vi "Solenoids_and_Deflection.vi"() -> ()   [LabVIEW 2018]
panel:
  out "?":string
  out "?":string
  out "?":string
  out "?":string
  in  "Set Agilent 2":bool
  out "?":bool
  out "?":bool
  out "?":string
  in  "Set Agilent":bool
  out "?":bool
  out "?":bool
  out "?":string
  out "Sensors":string
  # "Waveform:\nTriangle"
  # "Peak B-Field:\n90 G"
  # "Solenoid (M1)"
  # "Freq | Amp:\n20 Hz | 10 V"
  # "Peak Current:\n1.7 A"
  # "Solenoid (M2)"
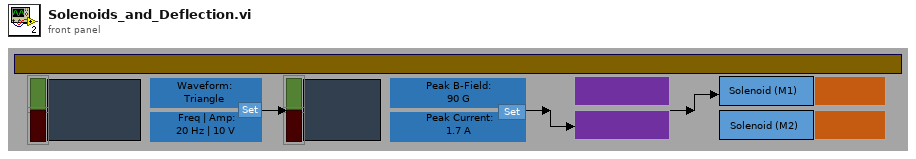
[diagram p1: front panel]
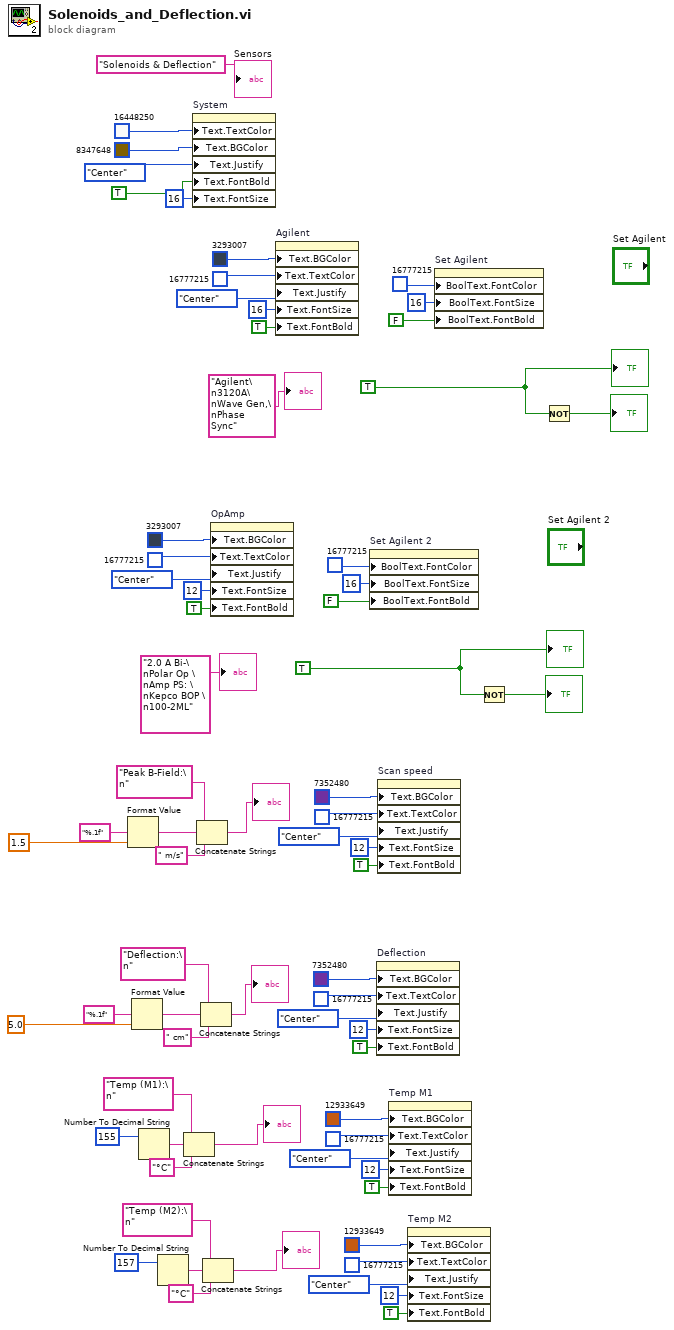
[diagram p0: block diagram]
diagram:
  w44 = TRUE
  w55 = TRUE
  n1 = Format Value(format string="%.1f", value (0)=1.5) -> (output string=w29:string)  [unwired: 1 in]
  n2 = Format Value(format string="%.1f", value (0)=5.0) -> (output string=w23:string)  [unwired: 1 in]
  n3 = Number To Decimal String(number=155) -> (decimal integer string=w14:string)  [unwired: 1 in]
  n4 = Number To Decimal String(number=157) -> (decimal integer string=w4:string)  [unwired: 1 in]
  n5 = Concatenate Strings("Temp (M1):\n", w14, "°C" ("string")) -> (→"?":string)
  n6 = property on="System" class="Str"("Text.TextColor"=u32 16448250, "Text.BGColor"=u32 8347648, "Text.Justify"=enum16{"Left", "Center", "Right"}."Center" ("Text.Justification"), "Text.FontBold"=TRUE ("Text.Font:Bold"), "Text.FontSize"=u32 16 ("Text.Font:Size")) -> ()  [unwired: 2 in, 2 out]
  n7 = Concatenate Strings("Peak B-Field:\n", w29, " m/s" ("string")) -> (→"?":string)
  n8 = Concatenate Strings("Deflection:\n", w23, " cm" ("string")) -> (→"?":string)
  n9 = Concatenate Strings("Temp (M2):\n", w4, "°C" ("string")) -> (→"?":string)
  n10 = property on="OpAmp" class="Str"("Text.BGColor"=u32 3293007, "Text.TextColor"=u32 16777215, "Text.Justify"=enum16{"Left", "Center", "Right"}."Center" ("Text.Justification"), "Text.FontSize"=u32 12 ("Text.Font:Size"), "Text.FontBold"=TRUE ("Text.Font:Bold")) -> ()  [unwired: 2 in, 2 out]
  n11 = property on="Agilent" class="Str"("Text.BGColor"=u32 3293007, "Text.TextColor"=u32 16777215, "Text.Justify"=enum16{"Left", "Center", "Right"}."Center" ("Text.Justification"), "Text.FontSize"=u32 16 ("Text.Font:Size"), "Text.FontBold"=TRUE ("Text.Font:Bold")) -> ()  [unwired: 2 in, 2 out]
  n12 = property on="Set Agilent 2" class="Bool (strict)"("BoolText.FontColor"=u32 16777215, "BoolText.FontSize"=u32 16 ("Boolean Text.Font:Size"), "BoolText.FontBold"=FALSE ("Boolean Text.Font:Bold")) -> ()  [unwired: 2 in, 2 out]
  n13 = property on="Deflection" class="Str"("Text.BGColor"=u32 7352480, "Text.TextColor"=u32 16777215, "Text.Justify"=enum16{"Left", "Center", "Right"}."Center" ("Text.Justification"), "Text.FontSize"=u32 12 ("Text.Font:Size"), "Text.FontBold"=TRUE ("Text.Font:Bold")) -> ()  [unwired: 2 in, 2 out]
  n14 = property on="Scan speed" class="Str"("Text.BGColor"=u32 7352480, "Text.TextColor"=u32 16777215, "Text.Justify"=enum16{"Left", "Center", "Right"}."Center" ("Text.Justification"), "Text.FontSize"=u32 12 ("Text.Font:Size"), "Text.FontBold"=TRUE ("Text.Font:Bold")) -> ()  [unwired: 2 in, 2 out]
  n15 = property on="Temp M1" class="Str"("Text.BGColor"=u32 12933649, "Text.TextColor"=u32 16777215, "Text.Justify"=enum16{"Left", "Center", "Right"}."Center" ("Text.Justification"), "Text.FontSize"=u32 12 ("Text.Font:Size"), "Text.FontBold"=TRUE ("Text.Font:Bold")) -> ()  [unwired: 2 in, 2 out]
  n16 = property on="Temp M2" class="Str"("Text.BGColor"=u32 12933649, "Text.TextColor"=u32 16777215, "Text.Justify"=enum16{"Left", "Center", "Right"}."Center" ("Text.Justification"), "Text.FontSize"=u32 12 ("Text.Font:Size"), "Text.FontBold"=TRUE ("Text.Font:Bold")) -> ()  [unwired: 2 in, 2 out]
  n17 = property on="Set Agilent" class="Bool (strict)"("BoolText.FontColor"=u32 16777215, "BoolText.FontSize"=u32 16 ("Boolean Text.Font:Size"), "BoolText.FontBold"=FALSE ("Boolean Text.Font:Bold")) -> ()  [unwired: 2 in, 2 out]
  n18 = Not(x=w44) -> (.not. x?=→"?":bool)
  n19 = Not(x=w55) -> (.not. x?=→"?":bool)
  "Sensors" <- "Solenoids & Deflection" ("Sensors")
  "?" <- "Agilent\n3120A\nWave Gen,\nPhase Sync"
  "?" <- w55
  "?" <- "2.0 A Bi-\nPolar Op \nAmp PS: \nKepco BOP \n100-2ML"
  "?" <- w44
